vi "GetContMeasData ohne Schleife.vi"(8 "error in (no error)":errorcluster, 10 "queue out":refnum<queue>, 11 "TCP Network Connection in":refnum<k5>) -> (0 "error out":errorcluster, 1 "Messabbruch":bool, 2 "Meas Result":dbl[](array[numeric]), 3 "TCP Network Connection out":refnum<k5>, 5 "Sonstige Nachrichten":string[](array[string]))   [LabVIEW 2017]
uses:
  AT901 API/TypeDefinitions/ES_DataType.ctl
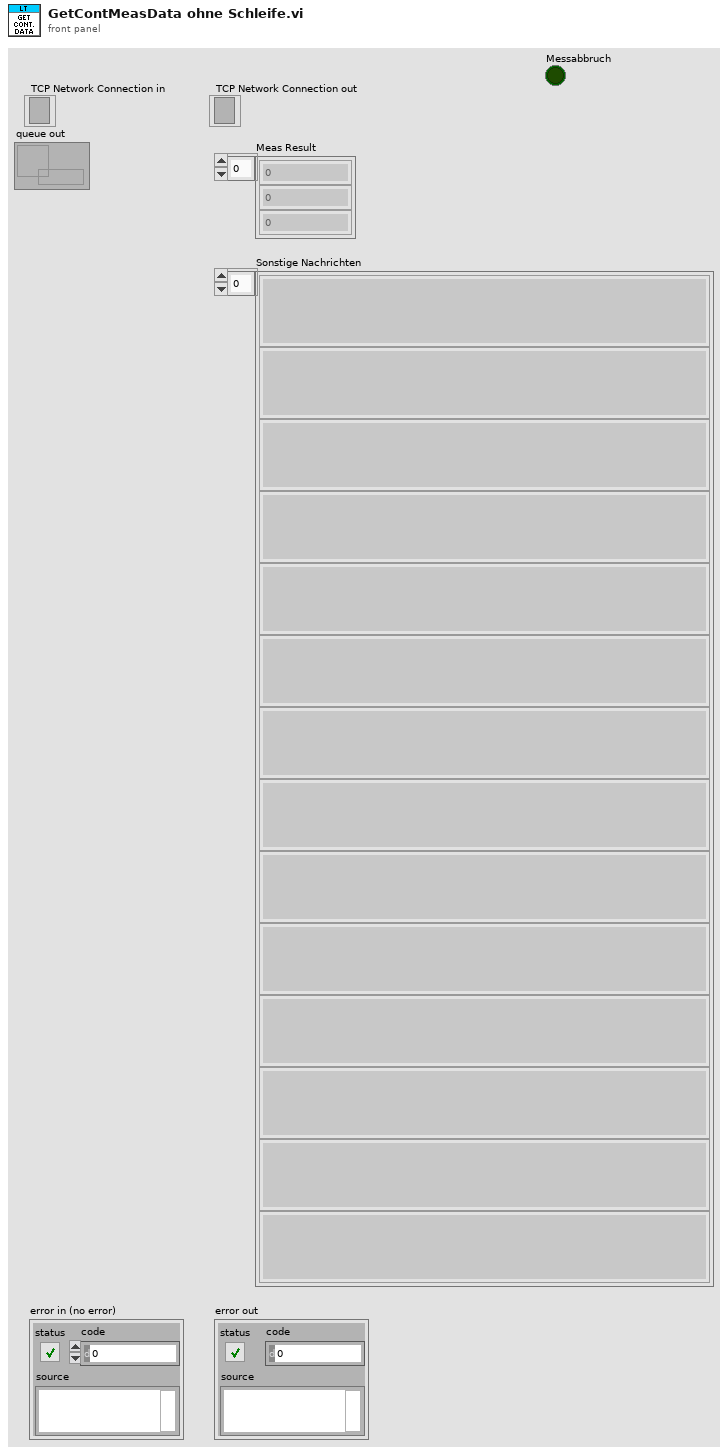
[diagram p1: front panel]
types:
  T1 = typedef "ES_DataType.ctl" = enum32{"ES_DT_Command", "ES_DT_Error", "ES_DT_SingleMeasResult", "ES_DT_MultiMeasResult", "ES_DT_StationaryProbeMeasResult", "ES_DT_ContinuousProbeMeasResult", "ES_DT_NivelResult", "ES_DT_ReflectorPosResult", "ES_DT_SystemStatusChange", "ES_DT_SingleMeasResult2", "ES_DT_MultiMeasResult2", "ES_DT_ProbePosResult"}
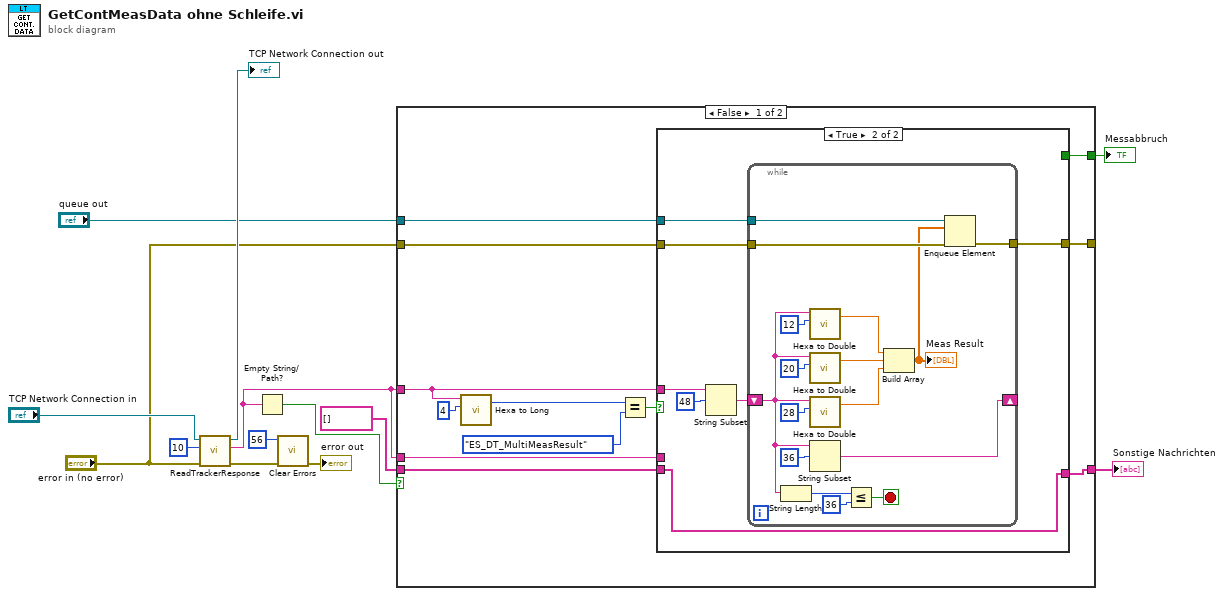
[diagram p0: block diagram]
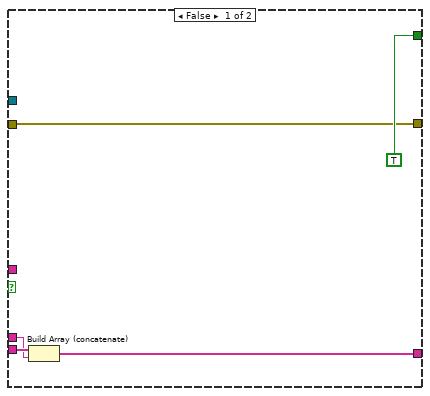
[diagram p2: hidden frame]
diagram:
  n1 = call "ReadTrackerResponse.vi"("error in"="error in (no error)", "timeout ms (1000)"=10, "connection ID in"="TCP Network Connection in") -> ("error out"=w8:errorcluster, "Tracker Response"=w5:string, "connection ID out"=→"TCP Network Connection out":refnum<k5>)  [unwired: 6 in]
  n2 = Empty String/Path?(string/path=w5) -> (empty?=w6:bool)
  n3 = call <vilib>:"Clear Errors.vi"("error in (no error)"=w8, "specific error code to clear (0: all)"=56) -> ("error out"=→"error out":errorcluster)  [unwired: 4 in, 1 out]
  n4 = case shown="False" w6 {
    tunnel: w5 -> [w21 _]
    tunnel: string[] [] -> [w20 w55]
    tunnel: w5 -> [w19 _]
    tunnel: [w18 w55] -> w12
    tunnel: [w17 _] -> w3
    tunnel: "queue out" -> [w16 _]
    tunnel: "error in (no error)" -> [w15 w54]
    tunnel: [w14 w54] -> _
    frame False {
      n5 = call "Hexa to Long.vi"("Hexa"=w21, "Index"=4) -> ("Long"=w24:u32)  [unwired: 4 in]
      n6 = Equal?(x=w24, y=ES_DataType."ES_DT_MultiMeasResult" ("ES_DataType")) -> (x = y?=w22:bool)
      n7 = case shown="True" w22 {
        tunnel: w21 -> [_ w35]
        tunnel: w20 -> [w30 w34]
        tunnel: w19 -> [w29 _]
        tunnel: [w28 w34] -> w18
        tunnel: [TRUE _] -> w17
        tunnel: w16 -> [_ w33]
        tunnel: w15 -> [w26 w32]
        tunnel: [w26 w31] -> w14
        frame False {
          n8 = Build Array (concatenate)(w30, w29) -> (w28:string[])
        }
        frame True {
          n9 = String Subset(string=w35, offset (0)=48) -> (substring=w36:string)  [unwired: 1 in]
          n10 = while {
            shift-right: [w42] -> _
            shift-left: w36 -> [w43]
            tunnel: w33 -> [w41]
            tunnel: w32 -> [w40]
            tunnel: [w39] -> w31
            stop <- w51 stop-if-true
            n11 = String Length(string=w43) -> (length=w53:i32)
            n12 = call "Hexa to Double.vi"("Hexa"=w43, "Index"=12) -> ("Double"=w50:dbl)  [unwired: 4 in]
            n13 = call "Hexa to Double.vi"("Hexa"=w43, "Index"=20) -> ("Double"=w49:dbl)  [unwired: 4 in]
            n14 = call "Hexa to Double.vi"("Hexa"=w43, "Index"=28) -> ("Double"=w48:dbl)  [unwired: 4 in]
            n15 = String Subset(string=w43, offset (0)=36) -> (substring=w42:string)  [unwired: 1 in]
            n16 = Less Or Equal?(x=w53, y=36) -> (x <= y?=w51:bool)
            n17 = Build Array(w50, w49, w48) -> (w38:dbl[])
            "Meas Result" <- w38
            n18 = Enqueue Element(queue=w41, element=w38, error in (no error)=w40) -> (error out=w39:errorcluster)  [unwired: 1 in, 2 out]
          }
        }
      }
    }
    frame True {
    }
  }
  "Sonstige Nachrichten" <- w12
  "Messabbruch" <- w3
